vi "Present Data.vi"(8 "error in (no error)":errorcluster, 11 "List Seen Processes View Model In":refnum<class "Multicolumn List Box View Model.lvclass">) -> (0 "error out":errorcluster, 2 "Data":string[][](array[string]), 3 "List Seen Processes View Model Out":refnum<class "Multicolumn List Box View Model.lvclass">)   [LabVIEW 2020, in "Multicolumn List Box View Model.lvclass"]
uses:
  Multicolumn List Box View Model.lvclass
  Multicolumn List Box View Model.lvclass/Multicolumn List Box View Model.ctl
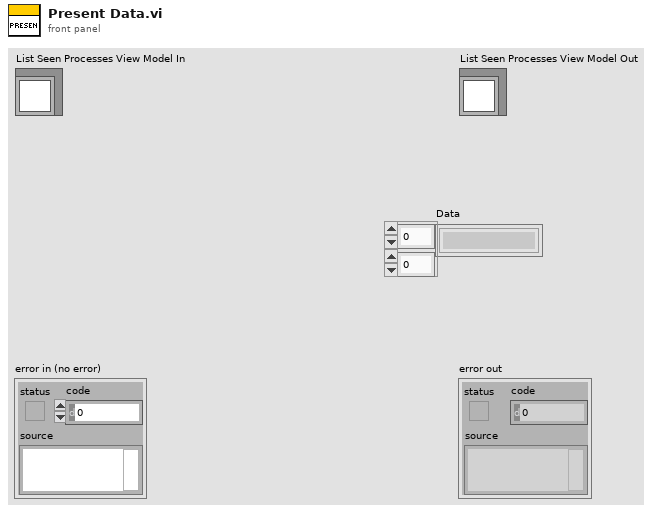
[diagram p1: front panel]
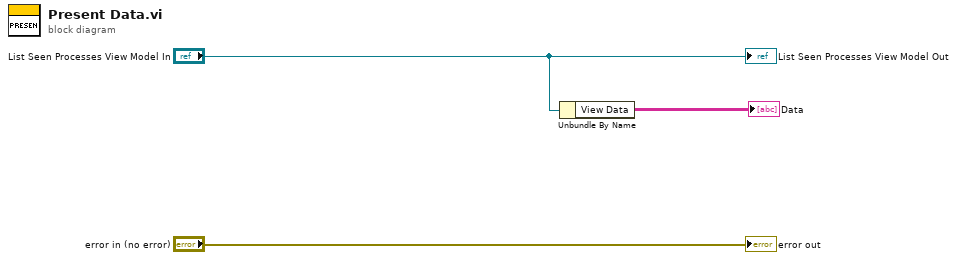
[diagram p0: block diagram]
diagram:
  n1 = Unbundle By Name("List Seen Processes View Model In") -> ("View Data"=→"Data":string[][])
  "error out" <- "error in (no error)"
  "List Seen Processes View Model Out" <- "List Seen Processes View Model In"
